vi "Actor Core.vi"(8 "error in":cluster{"状态":bool, "代码":i32, "源":string} caption="错误输入", 11 "气冷系统应用程序":refnum<class "Air Cooler Application.lvclass">) -> (0 "error out":cluster{"状态":bool, "代码":i32, "源":string} caption="错误输出", 3 "操作者输出":refnum<class "Actor.lvclass">)   [LabVIEW 2013, in "Air Cooler Application.lvlib" / "Air Cooler Application.lvclass"]
doc: "Actor Core.vi包含操作者的主要消息处理循环。操作者通常位于该循环中，在各种消息到达时对消息进行处理。如Do.vi消息返回任何错误，该循环将停止运行，错误代码43将被作为“无错误停止”的标准信号发送给调用方。如需更改上述行为，可在子孙类的Handle Error.vi中对该部分逻辑进行重写。"
uses:
  Air Cooler Application.lvclass
  <vilib>/ActorFramework/Actor/Actor.lvclass
  Cooler/Cooler/Cooler.lvclass
  Live User Controller/Live User Controller.lvclass
  <vilib>/ActorFramework/Actor/Actor.lvclass/Actor.ctl
  <vilib>/ActorFramework/Message Enqueuer/Message Enqueuer.lvclass/Message Enqueuer.ctl
  Air Cooler Application.lvclass/Air Cooler Application.ctl
  <vilib>/ActorFramework/Stop Msg/Stop Msg.lvclass/Stop Msg.ctl
  Programmatic Controller/Programmatic Controller.lvclass
  Swap Controllers Msg/Swap Controllers Msg.lvclass/Swap Controllers Msg.ctl
  Cooler Controller/Write Cooler Enqueuer Msg/Write Cooler Enqueuer Msg.lvclass/Write Cooler Enqueuer Msg.ctl
  Cooler/Write Controller Enqueuer Msg/Write Controller Enqueuer Msg.lvclass/Write Controller Enqueuer Msg.ctl
  <vilib>/ActorFramework/Message Enqueuer/Init from Existing Queue.vi
  <vilib>/ActorFramework/Message Enqueuer/Enqueue.vi
  <vilib>/ActorFramework/Message Enqueuer/Enqueue Critical.vi
  <vilib>/ActorFramework/Message Priority Queue/Priority Enqueue.vi
  <vilib>/ActorFramework/Message Enqueuer/Message Enqueuer.lvclass
  <vilib>/ActorFramework/Stop Msg/Stop Msg.lvclass
  Swap Controllers Msg/Swap Controllers Msg.lvclass
  Cooler Controller/Write Cooler Enqueuer Msg/Write Cooler Enqueuer Msg.lvclass
  Cooler/Write Controller Enqueuer Msg/Write Controller Enqueuer Msg.lvclass
panel:
  in  "DNL_Controller Selection":enum32{"UI Option 1", "UI Option 2"}(radio)
  in  "停止":bool
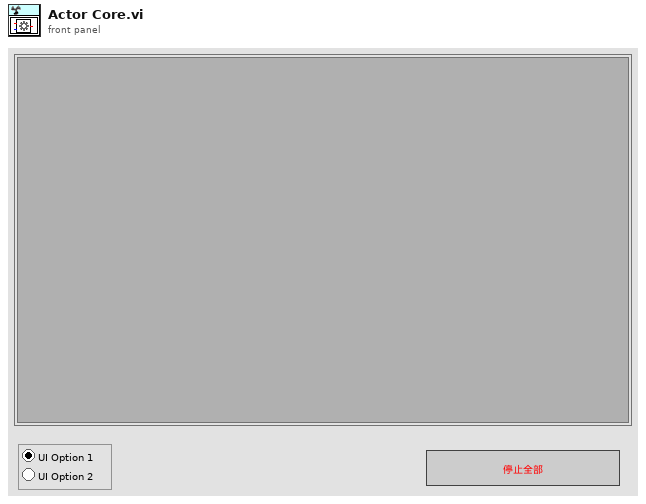
[diagram p1: front panel]
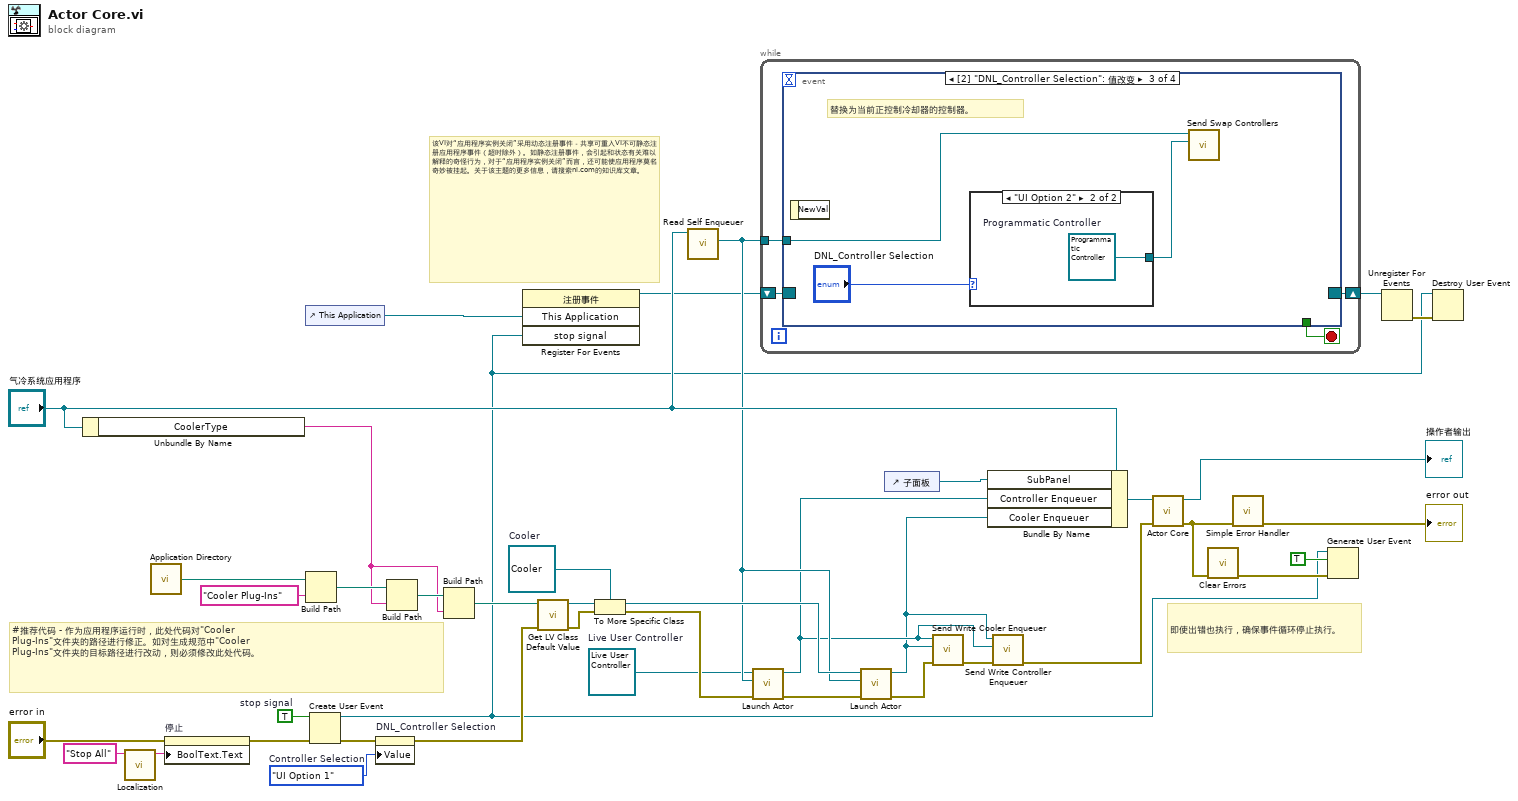
[diagram p0: block diagram]
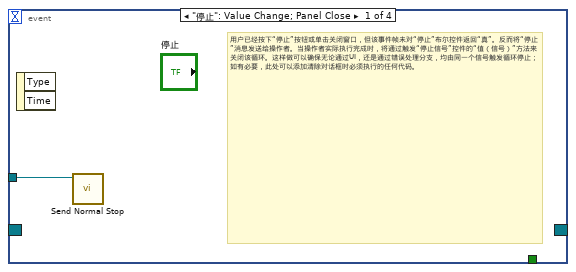
[diagram p2: hidden frame]
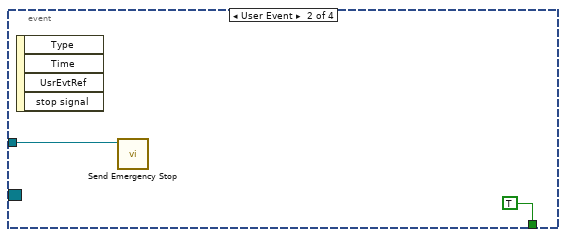
[diagram p3: hidden frame]
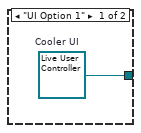
[diagram p4: hidden frame]
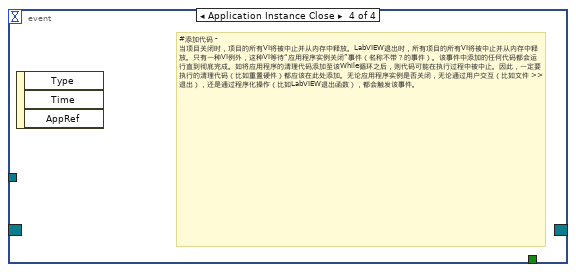
[diagram p5: hidden frame]
diagram:
  w1 = enum32{"UI Option 1", "UI Option 2"}."UI Option 1"  # Controller Selection
  w14 = TRUE  # stop signal
  w18 = refnum<class "Live User Controller.lvclass"> refnum  # Live User Controller
  w29 = refnum<class "Cooler.lvclass"> refnum  # Cooler
  # "该VI对“应用程序实例关闭”采用动态注册事件－共享可重入VI不可静态注册应用程序事件（超时除外）。如静态注册事件，会引起和状态有关难以解释的奇怪行为，对于“应用程序实例关闭”而言，还可能使应用程序莫名奇妙被挂起。关于该主题的更多信息，请搜索ni.com的知识库文章。"
  # "#推荐代码 - 作为应用程序运行时，此处代码对\"Cooler Plug-Ins\"文件夹的路径进行修正。如对生成规范中\"Cooler Plug-Ins\"文件夹的目标路径进行改动，则必须修改此处代码。"
  # "即使出错也执行，确保事件循环停止执行。"
  n1 = Unbundle By Name("气冷系统应用程序") -> ("CoolerType"=w20:string)
  n2 = call "Localization.vi"("未本地化"="Stop All" ("Unlocalized")) -> ("本地化"=w35:string)  [unwired: 10 in]
  n3 = call <vilib>:"Application Directory.vi"() -> ("Application Directory"=w2:path)
  n4 = property on="停止" class="Bool"(error in="error in", "BoolText.Text"=w35) -> (error out=w15:errorcluster)  [unwired: 1 in, 1 out]
  n5 = control-ref of="This Application"() -> (w3:refnum<vi>)
  n6 = Build Path(base path=w2, name or relative path="Cooler Plug-Ins") -> (appended path=w24:path)
  n7 = Create User Event(user event datatype=w14, error in=w15) -> (user event=w4:refnum<user-event>, error out=w8:errorcluster)
  n8 = property on="DNL_Controller Selection" class="RadioBtnsControl (严格)"(error in=w8, "Value"=w1) -> (error out=w7:errorcluster)  [unwired: 1 in, 1 out]
  n9 = Build Path(base path=w24, name or relative path=w20) -> (appended path=w33:path)
  n10 = Build Path(base path=w33, name or relative path=w20) -> (appended path=w32:path)
  n11 = register-events(w3, w4) -> (reference out=w13:refnum<event-registration>)  [unwired: 2 in, 1 out]
  n12 = call <vilib>:"Get LV Class Default Value.vi"("error in (no error)"=w7, "class path"=w32) -> ("error out"=w30:errorcluster, "object"=w31:refnum<class>)  [unwired: 8 in]
  n13 = To More Specific Class(target class=w29, reference=w31, error in=w30) -> (specific class reference=w28:refnum<class "Cooler.lvclass">, error out=w19:errorcluster)
  n14 = call <vilib>:"Read Self Enqueuer.vi"("Actor"="气冷系统应用程序") -> ("Self Enqueuer"=w23:refnum<class "Message Enqueuer.lvclass">)  [unwired: 10 in]
  n15 = call <vilib>:"Launch Actor.vi"("error in (no error)"=w19, "Actor-to-Caller Enqueuer"=w23, "Actor"=w18) -> ("error out"=w39:errorcluster, "Caller-To-Actor Enqueuer"=w17:refnum<class "Message Enqueuer.lvclass">)  [unwired: 7 in]
  n16 = while {
    tunnel: w23 -> [w44]
    shift-right: [w41] -> w10
    shift-left: w13 -> [w42]
    stop <- w43 stop-if-true
    n17 = event shown="[2] \"DNL_Controller Selection\": 值改变" {
      selector: w42 -> [_ _ _ _]
      dyn-events: [_ _ _ _] -> w41
      timeout: _ -> [_ _ _ _]
      tunnel: w44 -> [w45 w47 w50 _]
      tunnel: [_ TRUE _ _] -> w43
      event "停止": Value Change; Panel Close {
        # "用户已经按下“停止”按钮或单击关闭窗口，但该事件帧未对“停止”布尔控件返回“真”。反而将“停止”消息发送给操作者。当操作者实际执行完成时，将通过触发“停止信号”控件的“值（信号）”方法来关闭该循环。这样做可以确保无论通过UI，还是通过错误处理分支，均由同一个信号触发循环停止；如有必要，此处可以添加清除对话框时必须执行的任何代码。"
        n18 = event-data() -> ()  [unwired: 1 in, 2 out]
        n19 = call <vilib>:"Send Normal Stop.vi"("Message Enqueuer"=w45) -> ()  [unwired: 10 in, 1 out]
      }
      event User Event {
        n20 = event-data() -> ()  [unwired: 1 in, 4 out]
        n21 = call <vilib>:"Send Emergency Stop.vi"("Message Enqueuer"=w47) -> ()  [unwired: 10 in, 1 out]
      }
      event "DNL_Controller Selection": Value Change {
        # "替换为当前正控制冷却器的控制器。"
        n22 = event-data() -> ()  [unwired: 1 in, 1 out]
        n23 = case shown="\"UI Option 2\"" "DNL_Controller Selection" {
          tunnel: [w51 w52] -> w48
          frame "UI Option 1" {
            w51 = refnum<class "Live User Controller.lvclass"> refnum  # Cooler UI
          }
          frame "UI Option 2" {
            w52 = refnum<class "Programmatic Controller.lvclass"> refnum  # Programmatic Controller
          }
        }
        n24 = call "Send Swap Controllers.vi"("冷却器控制器"=w48, "消息待入队列"=w50) -> ()  [unwired: 9 in, 1 out]
      }
      event Application Instance Close {
        # "#添加代码 - 当项目关闭时，项目的所有VI将被中止并从内存中释放。LabVIEW退出时，所有项目的所有VI将被中止并从内存中释放。只有一种VI例外，这种VI等待“应用程序实例关闭”事件（名称不带？的事件）。该事件中添加的任何代码都会运行直到彻底完成。如将应用程序的清理代码添加至该While循环之后，则代码可能在执行过程中被中止。因此，一定要执行的清理代码（比如重置硬件）都应该在此处添加。无论应用程序实例是否关闭，无论通过用户交互（比如文件 >> 退出），还是通过程序化操作（比如LabVIEW退出函数），都会触发该事件。"
        n25 = event-data() -> ()  [unwired: 1 in, 3 out]
      }
    }
  }
  n26 = call <vilib>:"Launch Actor.vi"("error in (no error)"=w39, "Actor-to-Caller Enqueuer"=w23, "Actor"=w28) -> ("error out"=w26:errorcluster, "Caller-To-Actor Enqueuer"=w16:refnum<class "Message Enqueuer.lvclass">)  [unwired: 7 in]
  n27 = control-ref of="子面板"() -> (w27:refnum<vi>)
  n28 = call "Send Write Cooler Enqueuer.vi"("error in (no error)"=w26, "冷却器待入队列"=w16, "消息待入队列"=w17) -> ("error out"=w22:cluster{"状态":bool, "代码":i32, "源":string})  [unwired: 8 in]
  n29 = Bundle By Name(cluster="气冷系统应用程序", "SubPanel"=w27, "Controller Enqueuer"=w17, "Cooler Enqueuer"=w16) -> (w38:refnum<class "Air Cooler Application.lvclass">)
  n30 = call "Send Write Controller Enqueuer.vi"("error in (no error)"=w22, "控制器待入队列"=w17, "消息待入队列"=w16) -> ("error out"=w21:cluster{"状态":bool, "代码":i32, "源":string})  [unwired: 8 in]
  n31 = call-parent "Actor Core.vi"("error in"=w21, "Actor in"=w38) -> ("error out"=w6:errorcluster, "Actor out"=→"操作者输出":refnum<class "Actor.lvclass">)  [unwired: 8 in]
  n32 = call <vilib>:"Clear Errors.vi"("error in (no error)"=w6) -> ("error out"=w12:errorcluster)  [unwired: 6 in]
  n33 = call <vilib>:"Simple Error Handler.vi"("error in (no error)"=w6) -> ("error out"=→"error out":errorcluster)  [unwired: 4 in, 4 out]
  n34 = Generate User Event(user event=w4, event data cluster=TRUE ("stop"), error in=w12) -> ()  [unwired: 1 in, 2 out]
  n35 = Unregister For Events(event registration refnum=w10) -> (error out=w9:errorcluster)  [unwired: 1 in]
  n36 = Destroy User Event(user event=w4, error in=w9) -> ()  [unwired: 1 out]
